vi "measureSupply.vi"(0 "Supply instrument handle":refnum<k15>, 1 "Supply Channel":string caption="Supply Chanel", 2 "Messdauer/ms":i32=5, 3 "error in (no error)":errorcluster) -> (5 "Supply Output":T1 {"Current mean" format="%0.2f"; "Voltage mean" format="%0.2f"}, 7 "Supply instrument handle":refnum<k15>, 8 "Supply Voltage":waveform(dbl), 9 "Supply Current":waveform(dbl), 10 "error out":errorcluster)   [LabVIEW 2018]
doc: "Als Supply kann die 4130 und die 4110 verwendet werden.\nDas Vi führt eine Spannungs/Strommessung über einen zu bestimmenden Zeitraum durch. \nAußerdem werden die min und MaxWerte aller gemessener Signale ermittelt.\nAbhängig von der Sample to Average Einstellung wird die Anzahl der Messungen bestimmt.\n\nDer Strom und Spannung wird als Zeitverlauf aufgezeichet. \nAußerdem können die Min und Max sowie die Durchschnittswerte ausgegeben werden. \n\nWird eine zu kleineMessdauer angegeben, so erfolgt trotzdem eine Messung.\nMessauer==0-->keine Messung\n\nKull 21.04.2016"
uses:
  Type/SupplyOutput.ctl
panel:
  out "Measurement:Samples To Average":i32
  out "Elapsed Time (s) 2":dbl caption="Verstrichene Zeit (s)"
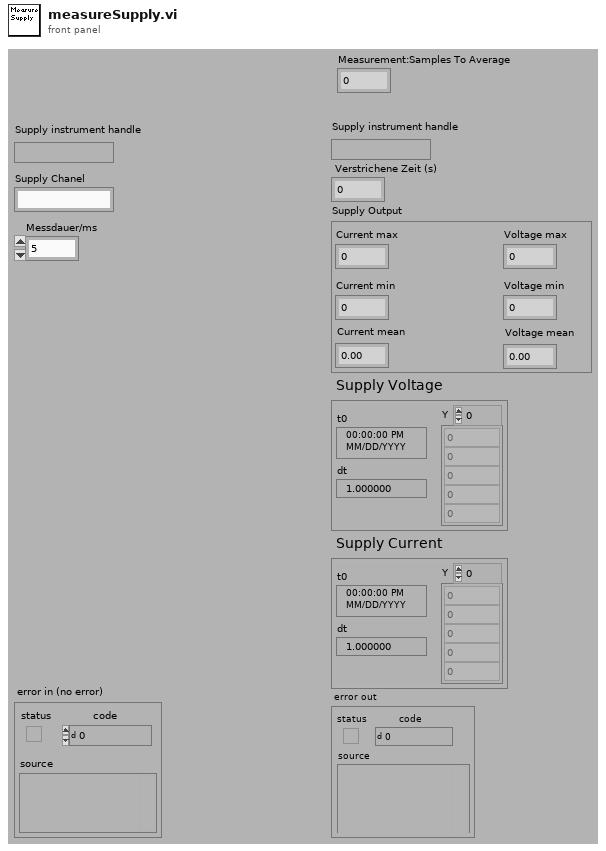
[diagram p1: front panel]
types:
  T1 = typedef "SupplyOutput.ctl" = cluster{"Current max":dbl, "Current min":dbl, "Voltage max":dbl, "Voltage min":dbl, "Voltage mean":dbl, "Current mean":dbl}
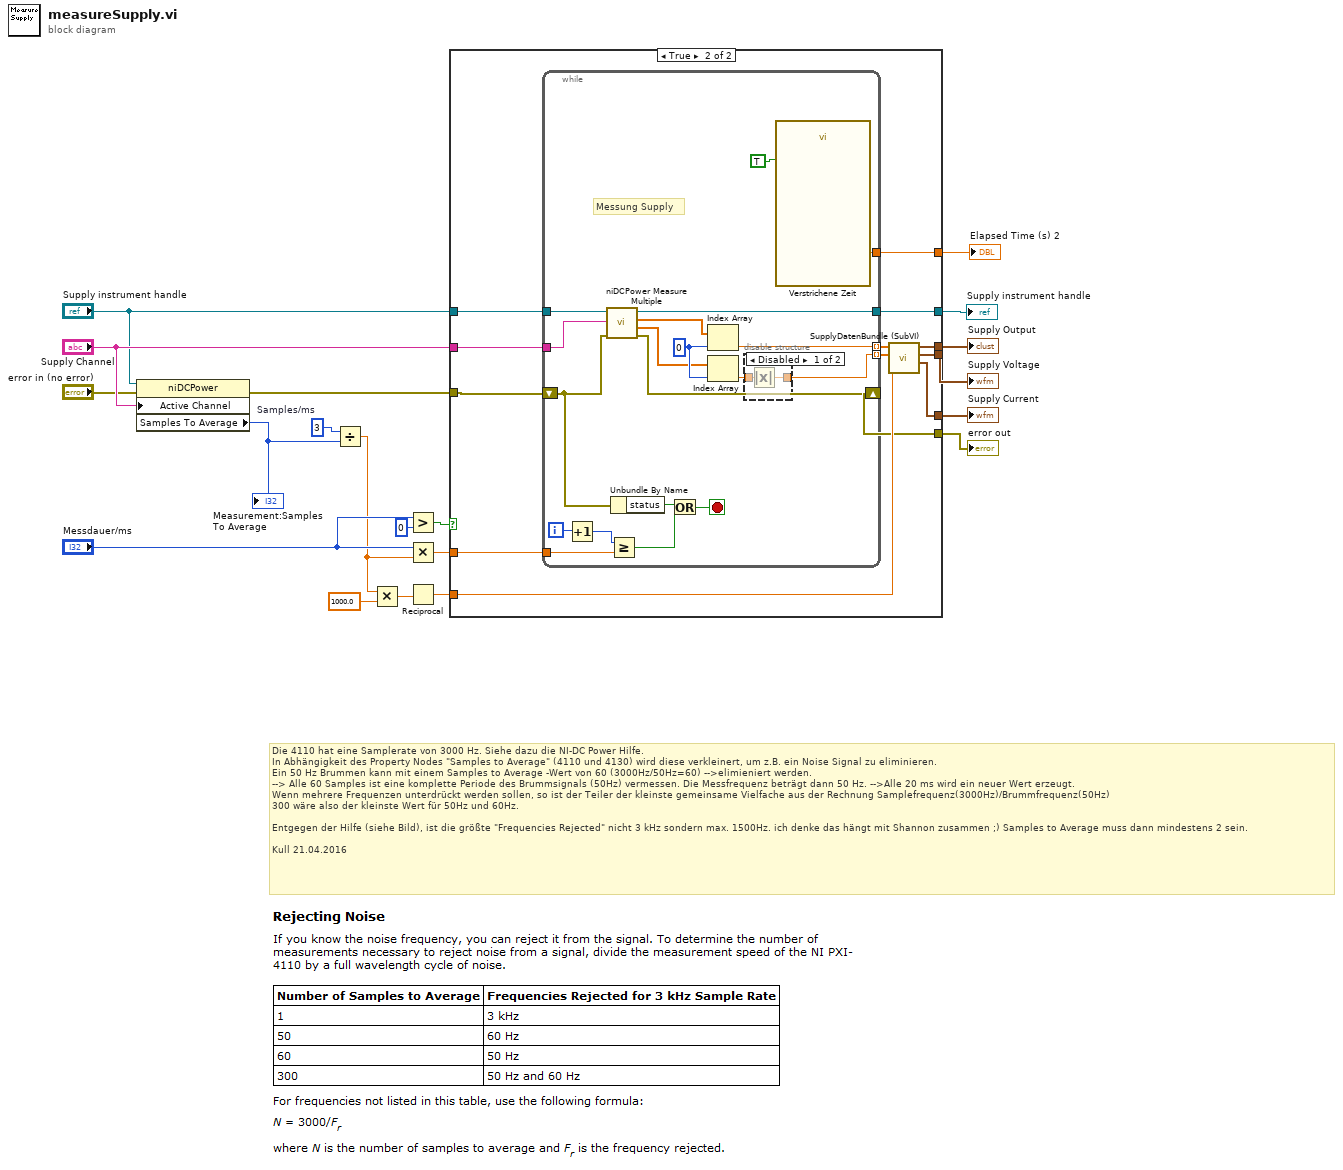
[diagram p0: block diagram]
diagram:
  w12 = 3  # Samples/ms
  # "Die 4110 hat eine Samplerate von 3000 Hz. Siehe dazu die NI-DC Power Hilfe.\nIn Abhängigkeit des Property Nodes \"Samples to Average\" (4110 und 4130) wird diese verkleinert, um z.B. ein Noise Signal zu eliminieren.\nEin 50 Hz Brummen kann mit einem Samples to Average -Wert von 60 (3000Hz/50Hz=60) -->elimieniert werden.\n--> Alle 60 Samples ist eine komplette Periode des Brummsignals (50Hz) vermessen. Die Messfrequenz beträgt dann 50 Hz. -->Alle 20 ms wird ein neuer Wert erzeugt.\nWenn mehrere Frequenzen unterdrückt werden sollen, so ist der Teiler der kleinste gemeinsame Vielfache aus der Rechnung Samplefrequenz(3000Hz)/Brummfrequenz(50Hz)\n300 wäre also der kleinste Wert für 50Hz und 60Hz.\n\nEntgegen der Hilfe (siehe Bild), ist die größte \"Frequencies Rejected\" nicht 3 kHz sondern max. 1500Hz. ich denke das hängt mit Shannon zusammen ;) Samples to Average muss dann mindestens 2 sein. \n\nKull 21.04.2016"
  n1 = property class="niDCPower"(reference="Supply instrument handle", error in="error in (no error)", "Active Channel"="Supply Channel") -> (error out=w8:errorcluster, "Samples To Average"=w11:i32)  [unwired: 1 out]
  "Measurement:Samples To Average" <- w11
  n2 = Divide(x=w12, y=w11) -> (x/y=w3:dbl)
  n3 = Multiply(x=w3, y=1000.0) -> (x*y=w4:dbl)
  n4 = Greater?(x="Messdauer/ms", y=0) -> (0:w5:bool)
  n5 = Multiply(x="Messdauer/ms", y=w3) -> (x*y=w20:dbl)
  n6 = Reciprocal(x=w4) -> (1/x=w16:dbl)
  n7 = case shown="True" w5 {
    tunnel: w20 -> [_ w23]
    tunnel: [_ w35] -> w19
    tunnel: [w21 w24] -> w18
    tunnel: [_ w34] -> w17
    tunnel: w16 -> [_ w33]
    tunnel: [_ w32] -> w15
    tunnel: [_ w31] -> w14
    tunnel: [w22 w28] -> w13
    tunnel: "Supply instrument handle" -> [w22 w27]
    tunnel: "Supply Channel" -> [_ w26]
    tunnel: w8 -> [w21 w25]
    frame False {
    }
    frame True {
      n8 = while {
        tunnel: w23 -> [w54]
        tunnel: [w53] -> w35
        tunnel: w27 -> [w52]
        tunnel: w26 -> [w51]
        tunnel: [w50] -> w28
        tunnel: [w49] -> w29 mode=indexing
        tunnel: [w48] -> w30 mode=indexing
        shift-right: [w43] -> w24
        shift-left: w25 -> [w44]
        i -> [w37]
        stop <- w42 stop-if-true
        w41 = 0 ("index")
        # "Messung Supply"
        n9 = Increment(x=w37) -> (x+1=w36:i32)
        n10 = call <instrlib>:"niDCPower Measure Multiple.vi"("error in (no error)"=w44, "channel name"=w51, "instrument handle"=w52) -> ("error out"=w43:errorcluster, "current measurements"=w40:dbl[], "voltage measurements"=w39:dbl[], "instrument handle out"=w50:refnum<k15>)  [unwired: 5 out]
        n11 = Greater Or Equal?(x=w36, y=w54) -> (x >= y?=w45:bool)
        n12 = Unbundle By Name(w44) -> ("status"=w46:bool)
        n13 = Or(x=w46, y=w45) -> (x .or. y?=w42:bool)
        n14 = Index Array(array=w39, index=w41) -> (element=w48:dbl)
        n15 = Index Array(array=w40, index=w41) -> (element=w38:dbl)
        n16 = disable-structure shown="Disabled" {
          disable-tunnel: [w56 w57] -> w49
          disable-tunnel: w38 -> [w55 w57]
          frame Disabled {
            n17 = Absolute Value(x=w55) -> (abs(x)=w56:dbl)
          }
          frame Enabled {
          }
        }
        n18 = call "Verstrichene Zeit"("Auto Reset"=TRUE) -> ("Elapsed Time (s)"=w53:dbl)  [unwired: 11 in, 7 out]
      }
      n19 = call "SupplyDatenBundle (SubVI).vi"("dt"=w33, "SupplyStrom"=w29, "SupplySpannung"=w30) -> ("Supply Current"=w32:waveform(dbl), "Supply Voltage"=w31:waveform(dbl), "Supply Output"=w34:T1)  [unwired: 6 in]
    }
  }
  "error out" <- w18
  "Elapsed Time (s) 2" <- w19
  "Supply Voltage" <- w14
  "Supply Current" <- w15
  "Supply Output" <- w17
  "Supply instrument handle" <- w13
